vi "Read Parameters to process.vi"(8 "error in":errorcluster, 11 "AppStateMachine runtime in":refnum<class "AppStateMachine runtime.lvclass">) -> (0 "error out":errorcluster, 2 "Parameters to process":T1, 3 "AppStateMachine runtime out":refnum<class "AppStateMachine runtime.lvclass">)   [LabVIEW 2017, in "AppStateMachine runtime.lvclass"]
uses:
  AppStateMachine runtime.lvclass
  configuration/parameter data indices.ctl
  AppStateMachine runtime.lvclass/AppStateMachine runtime.ctl
  configuration/AppStateMachine configuration.lvclass
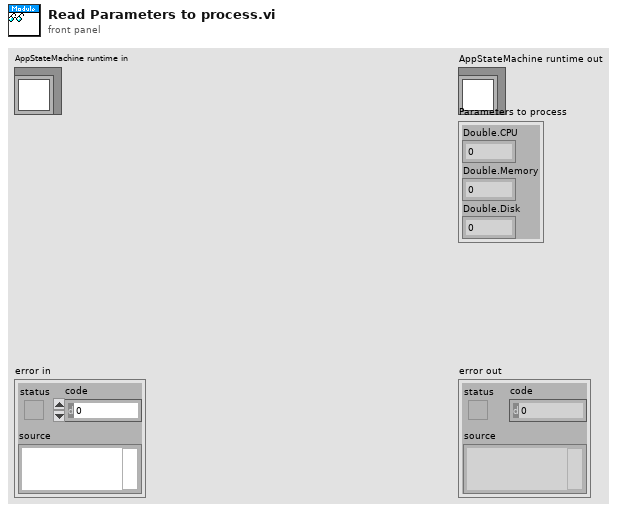
[diagram p1: front panel]
types:
  T1 = typedef "AppStateMachine configuration.lvclass/parameter data indices.ctl" = cluster{"Double.CPU":i32, "Double.Memory":i32, "Double.Disk":i32}
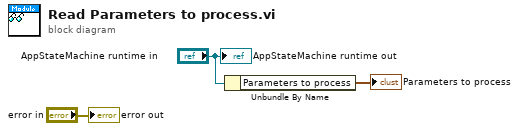
[diagram p0: block diagram]
diagram:
  n1 = Unbundle By Name("AppStateMachine runtime in") -> ("Parameters to process"=→"Parameters to process":T1)
  "error out" <- "error in"
  "AppStateMachine runtime out" <- "AppStateMachine runtime in"
